vi "get_minimum_and_maximum.vi"(8 "error in (no error)":errorcluster, 11 "Box in":refnum<class "Box.lvclass">) -> (0 "error out":errorcluster, 1 "maximum":refnum<class "SpaceVector.lvclass">, 2 "minimum":refnum<class "SpaceVector.lvclass">, 3 "Box out":refnum<class "Box.lvclass">)   [LabVIEW 2010, in "Box.lvclass"]
uses:
  Box.lvclass
  SpaceVector/SpaceVector/SpaceVector.lvclass
  Box.lvclass/Box.ctl
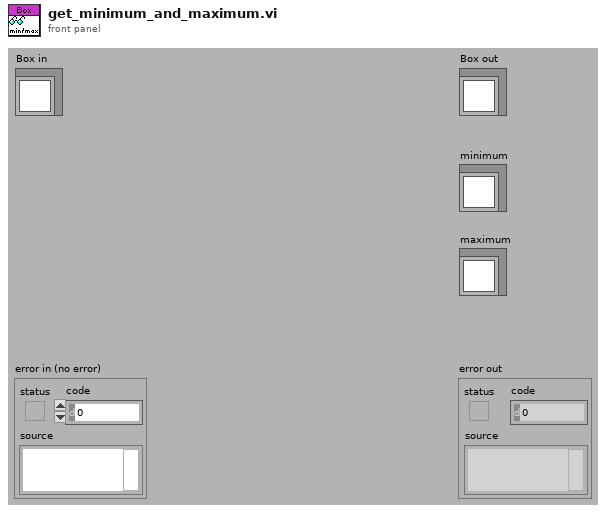
[diagram p1: front panel]
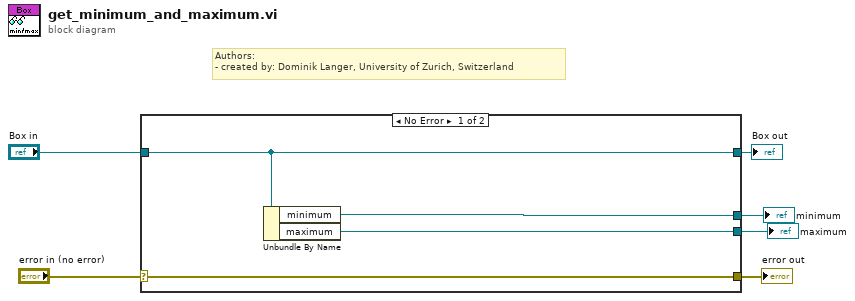
[diagram p0: block diagram]
diagram:
  # "Authors: \n- created by: Dominik Langer, University of Zurich, Switzerland"
  n1 = case shown="No Error" "error in (no error)" {
    selector: "error in (no error)" -> [w10 w12]
    tunnel: [w10 w12] -> w5
    tunnel: [w9 w11] -> w3
    tunnel: "Box in" -> [w9 w11]
    tunnel: [w8 _] -> w2
    tunnel: [w7 _] -> w1
    frame No Error {
      n2 = Unbundle By Name(w9) -> ("minimum"=w8:refnum<class "SpaceVector.lvclass">, "maximum"=w7:refnum<class "SpaceVector.lvclass">)
    }
    frame Error {
    }
  }
  "error out" <- w5
  "Box out" <- w3
  "minimum" <- w2
  "maximum" <- w1
